vi "Autonomous_Load.vi"(0 "Number of Commands":i32, 5 "Subsystems":string[](array[string]), 7 "Commands":string[](array[string]), 9 "Inputs":string[][](array[string]), 11 "error in":errorcluster) -> (4 "Queue_Key":refnum<queue>, 10 "Autonomous_Queue":refnum<queue>, 15 "errror out":errorcluster)   [LabVIEW 2018]
uses:
  Autonomous Utilities/Queue_Key_Data.ctl
  Autonomous Utilities/Robot_Subsystems.ctl
  Subsytems/Drive/Drive_Notifier.ctl
  Subsytems/Drive/Drive_Control_Type.ctl
  Subsytems/Elevator/Elevator_Notifier.ctl
  Subsytems/Elevator/Elevator_Control_Type.ctl
  Subsytems/Elevator/Elevator_Enum_States.ctl
  Subsytems/Climb/Climb_Notifier.ctl
  Subsytems/Climb/Climb_Control_Type.ctl
  Subsytems/Intake_Ball/Intake_Ball_Notifier.ctl
  Subsytems/Intake_Ball/Intake_Ball_Control_Type.ctl
  Subsytems/Intake_Disc/Intake_Disc_Notifier.ctl
  Subsytems/Intake_Disc/Intake_Disc_Control_Type.ctl
  <vilib>/Rock Robotics/WPI/Solenoid/WPI_SolenoidValue.ctl
  Subsytems/Intake_Joint/Intake_Joint_Notifier.ctl
  Subsytems/Intake_Joint/Intake_Joint_Control_Type.ctl
  Subsytems/Intake_Joint/Intake_Joint_Enum_States.ctl
panel:
  in  "Intake_Disc_Control_Type":T1
  in  "Intake_Ball_Control_Type":T2
  in  "Set Position":T3=enum."High_Rocket_Hatch_Panel_Floor"
  in  "Intake_Joint_Control_Type":T4
  in  "Set_Position":T5=enum."High_Rocket_Hatch_Panel_Floor"
  in  "Elevator_Control_Type":T6
  in  "Climb_Control_Type":T7
  in  "Drive_Control_List":T8=enum."Write_FL_Position"
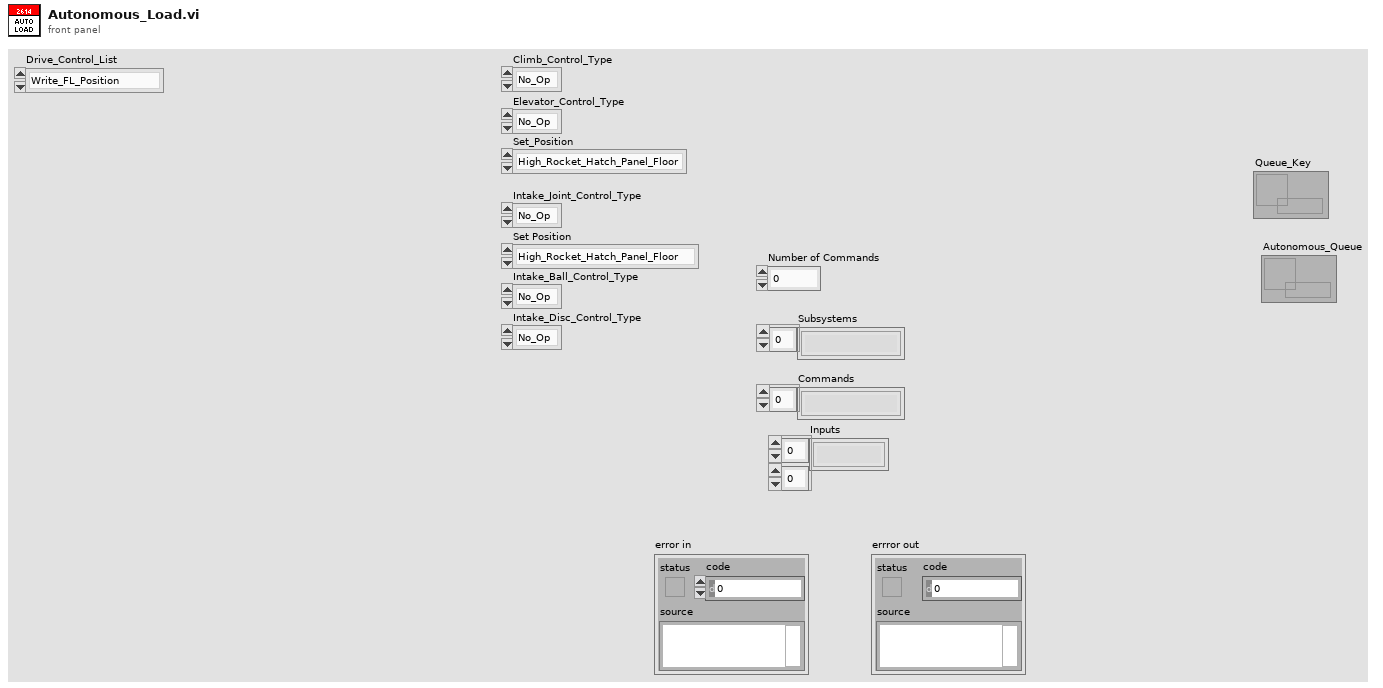
[diagram p1: front panel]
types:
  T1 = typedef "Intake_Disc_Control_Type.ctl" = enum16{"No_Op", "Manual_Disc_Toggle", "Disc_Toggle", "Manual_Press_Toggle", "Press_Toggle", "Acquire_Hatch", "Retract"}
  T2 = typedef "Intake_Ball_Control_Type.ctl" = enum16{"No_Op", "Manual_In", "Manual_Out", "In_Sensor_Stop", "Out_Teleop", "Out", "Stall"}
  T3 = typedef "Intake_Joint_Enum_States.ctl" = enum16{"Current_Position", "High_Rocket_Hatch_Panel_Floor", "High_Rocket_Hatch_Panel", "Mid_Rocket_Hatch_Panel_Floor", "Mid_Rocket_Hatch_Panel", "Low_Rocket_Hatch_Panel", "Cargo_Ship_Hatch_Panel", "Loading_Station_Hatch_Panel", "Ground_Pickup_Hatch_Panel", "High_Rocket_Cargo", "Mid_Rocket_Cargo", "Low_Rocket_Cargo", "Cargo_Ship_Cargo", "Loading_Station_Cargo", "Ground_Pickup_Cargo", "Depot_Pickup_Cargo", "Stow_Cargo", "Get_Hatch"}
  T4 = typedef "Intake_Joint_Control_Type.ctl" = enum16{"No_Op", "Manual_Joint_Up", "Manual_Joint_Down", "Manual_Position_Control", "Position_Control", "Position"}
  T5 = typedef "Elevator_Enum_States.ctl" = enum16{"Current_Position", "High_Rocket_Hatch_Panel_Floor", "High_Rocket_Hatch_Panel", "Mid_Rocket_Hatch_Panel_Floor", "Mid_Rocket_Hatch_Panel", "Low_Rocket_Hatch_Panel", "Cargo_Ship_Hatch_Panel", "Loading_Station_Hatch_Panel", "Ground_Pickup_Hatch_Panel", "High_Rocket_Cargo", "Mid_Rocket_Cargo", "Low_Rocket_Cargo", "Cargo_Ship_Cargo", "Loading_Station_Cargo", "Ground_Pickup_Cargo", "Depot_Pickup_Cargo", "Descend_Off_Platform", "Stow_Cargo"}
  T6 = typedef "Elevator_Control_Type.ctl" = enum16{"No_Op", "Shift", "Brake", "Manual_Elevator_Up", "Manual_Elevator_Down", "Manual_Climb_Up", "Manual_Climb_Down", "Manual_Position_Control", "Elevator_Retract", "Elevator_Extend", "Brake_In_Climb", "Position_Control", "Position", "Shift_Climb"}
  T7 = typedef "Climb_Control_Type.ctl" = enum16{"No_Op", "Brake", "Manual_Climb_Up", "Manual_Climb_Down", "Manual_Drive_Forward", "Manual_Drive_Backward", "Back_Wheels_Forward", "Lift_Retract", "Lift_Extend", "Extend_to_Second_Level", "Spin"}
  T8 = typedef "Drive_Control_Type.ctl" = enum16{"No_Op", "Write_FL_Position", "Write_FR_Position", "Write_BL_Position", "Write_BR_Position", "Set_Encoder_Positions", "Fieldcentric_PercentVBus", "Fieldcentric", "Robotcentric", "Reset_Gyro", "FR_Wheel", "FL_Wheel", "BR_Wheel", "BL_Wheel", "Drive_Onto_Platform", "Manual_Wheel_Control", "Distance", "Turn_To_Heading", "Turn_To_Target", "Drive_To_Target", "Zero", "Auto_Target", "Drive_Over_Platform", "Heading_Lock", "Time"}
  T9 = typedef "Queue_Key_Data.ctl" = cluster{"Operation Notifier":refnum<notifier>, "Subsystem":string, "Concurrent":bool}
  T10 = typedef "Robot_Subsystems.ctl" = cluster{"Drive Notifier":T11, "Elevator_Notifier":T12, "Climb_Notifier":T13, "Intake_Ball_Notifier":T14, "Intake_Disc_Notifier":T15, "Intake_Joint_Notifier":T17}
  T11 = typedef "Drive_Notifier.ctl" = cluster{"Drive Control List":T8, "Front/Back":dbl, "Left/Right":dbl, "Turn":dbl, "Test_Joy_Y":dbl, "Test_Joy_X":dbl, "Set Wheel Encoder Positions":bool, "Robotcentric":bool, "Reset Gyro":bool, "Rotate Front Right":bool, "Rotate Front Left":bool, "Rotate Back Right":bool, "Rotate Back Left":bool, "Write_Encoder_Positions":bool, "Climb_Advance":bool, "Parameter_One":dbl, "Parameter_Two":dbl, "Parameter_Three":dbl, "Parameter_Four":dbl, "Drive_Notifier":refnum<notifier>, "Step":i32, "Climb_Reverse":bool, "Auto_Target":bool}
  T12 = typedef "Elevator_Notifier.ctl" = cluster{"Elevator_Control_Type":T6, "Shift":bool, "Brake":bool, "Manual_Lift_Up":bool, "Manual_Lift_Down":bool, "Climb_Advance":bool, "Climb_Reverse":bool, "Low_Rocket":bool, "Mid_Rocket":bool, "High_Rocket":bool, "Cargo_Ship":bool, "Hatch_Floor":bool, "Cargo_Floor":bool, "HP_Hatch":bool, "HP_Cargo":bool, "Depot_Cargo":bool, "Stow":bool, "Set_Position":T5, "Intake_Mode":bool, "Climb_Distance":dbl, "Level_Two":bool, "Parameter_One":dbl, "Parameter_Two":dbl, "Parameter_Three":dbl, "Step":i32, "Elevator_Notifier":refnum<notifier>, "Brake_State":bool, "Shift_State":bool}
  T13 = typedef "Climb_Notifier.ctl" = cluster{"Climb_Control_Type":T7, "Brake":bool, "Manual_Climb_Up":bool, "Manual_Drive_Forward":bool, "Manual_Drive_Backward":bool, "Manual_Climb_Down":bool, "Climb_Advance":bool, "Climb_Reverse":bool, "Parameter_One":dbl, "Parameter_Two":dbl, "Parameter_Three":dbl, "Step":i32, "Climb_Notifier":refnum<notifier>, "Climb_Distance":dbl, "Level_Two":bool, "Brake_State":bool, "Toggle_Servo":bool}
  T14 = typedef "Intake_Ball_Notifier.ctl" = cluster{"Intake_Ball_Control_Type":T2, "Manual_In":bool, "Manual_Out":bool, "Ball_In":bool, "Ball_Out":bool, "Parameter_One":dbl, "Parameter_Two":dbl, "Parameter_Three":dbl, "Step":i32, "Ball_Notifier":refnum<notifier>}
  T15 = typedef "Intake_Disc_Notifier.ctl" = cluster{"Intake_Disc_Control_Type":T1, "Manual_Disc_Toggle":bool, "Disc_Toggle":bool, "Disc_Toggle_State":bool, "Manual_Press_Toggle":bool, "Disc_Press_State":bool, "Press_Toggle":bool, "Press_Pnuematic":T16, "Disc_Pnuematic":T16, "Disc_Notifier":refnum<notifier>, "Step":i32}
  T16 = typedef "WPI_SolenoidValue.ctl" = enum16{"Off", "On", "Forward", "Reverse"}
  T17 = typedef "Intake_Joint_Notifier.ctl" = cluster{"Intake_Joint_Control_Type":T4, "Manual_Joint_Up":bool, "Manual_Joint_Down":bool, "Low_Rocket":bool, "Mid_Rocket":bool, "High_Rocket":bool, "Cargo_Ship":bool, "Hatch_Floor":bool, "Cargo_Floor":bool, "HP_Hatch":bool, "HP_Cargo":bool, "Depot_Cargo":bool, "Stow":bool, "Intake_Mode":bool, "Set Position":T3, "Parameter_One":dbl, "Parameter_Two":dbl, "Parameter_Three":dbl, "Step":i32, "Joint_Notifier":refnum<notifier>}
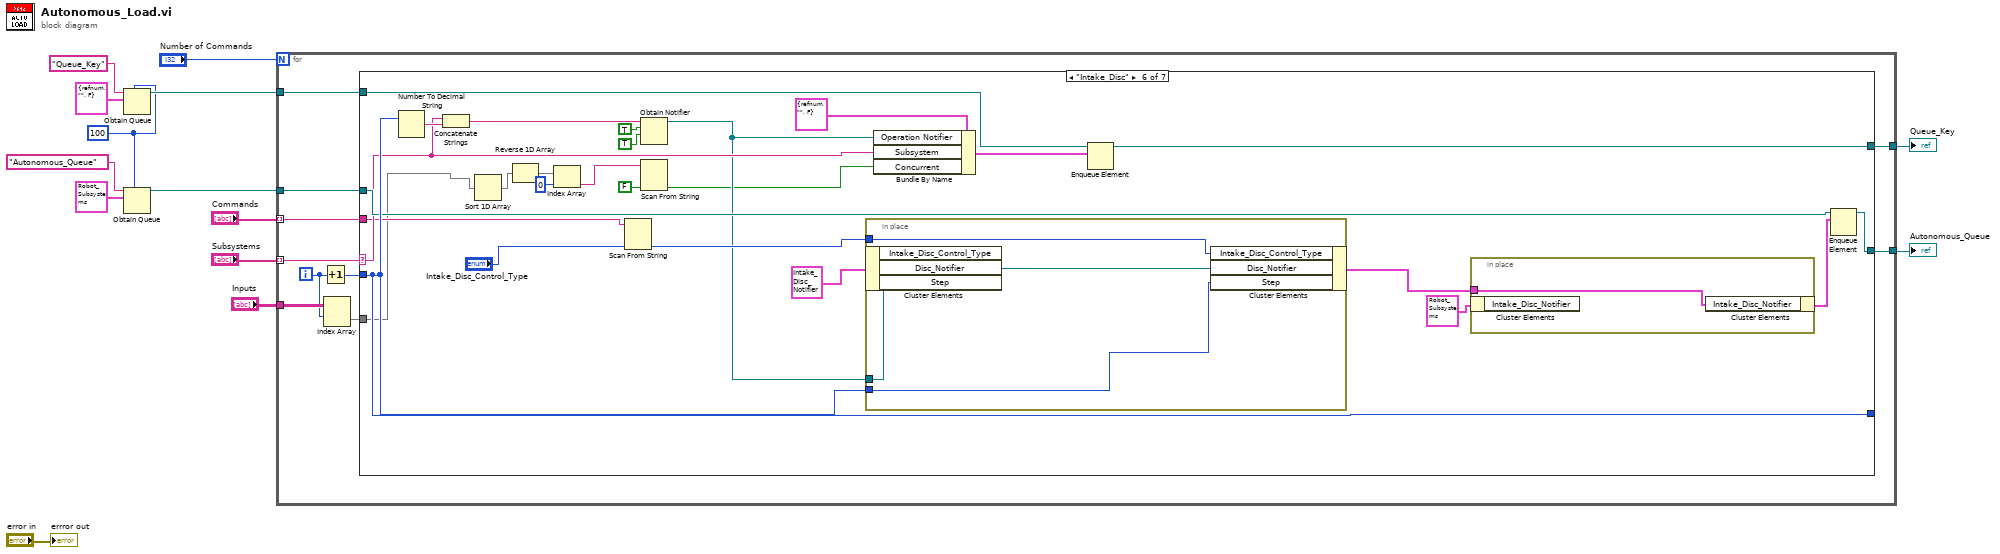
[diagram p0: block diagram]
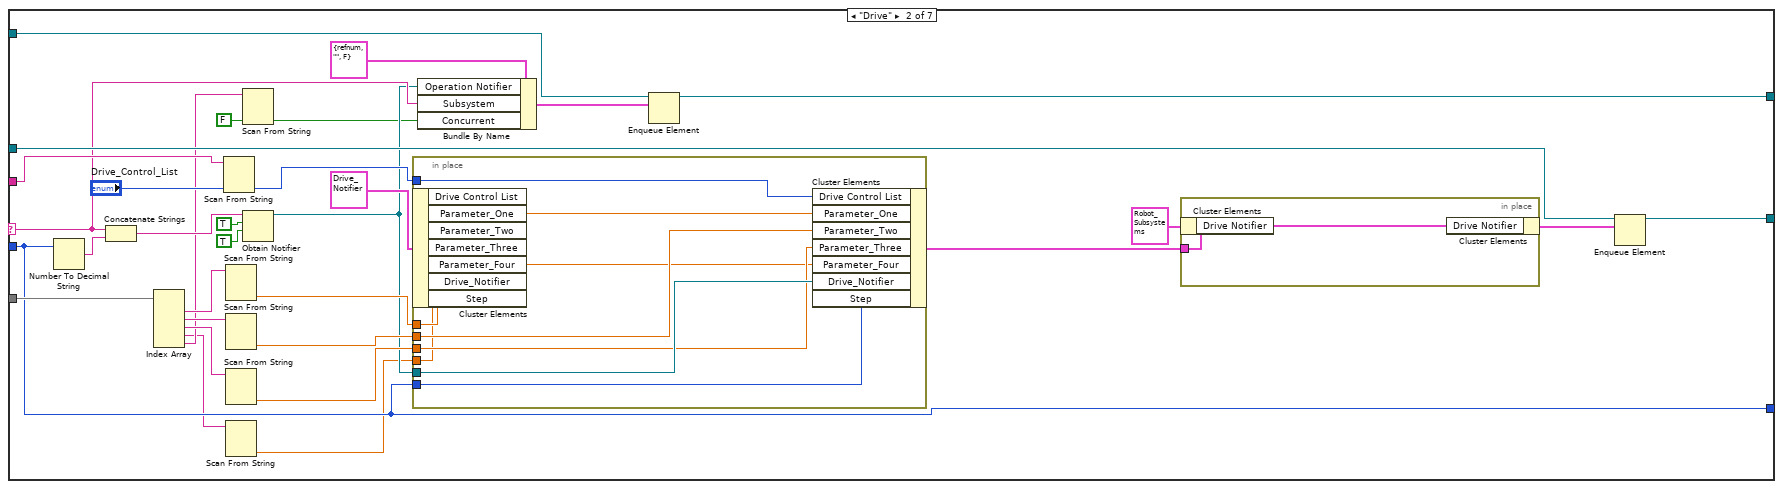
[diagram p3: hidden frame]
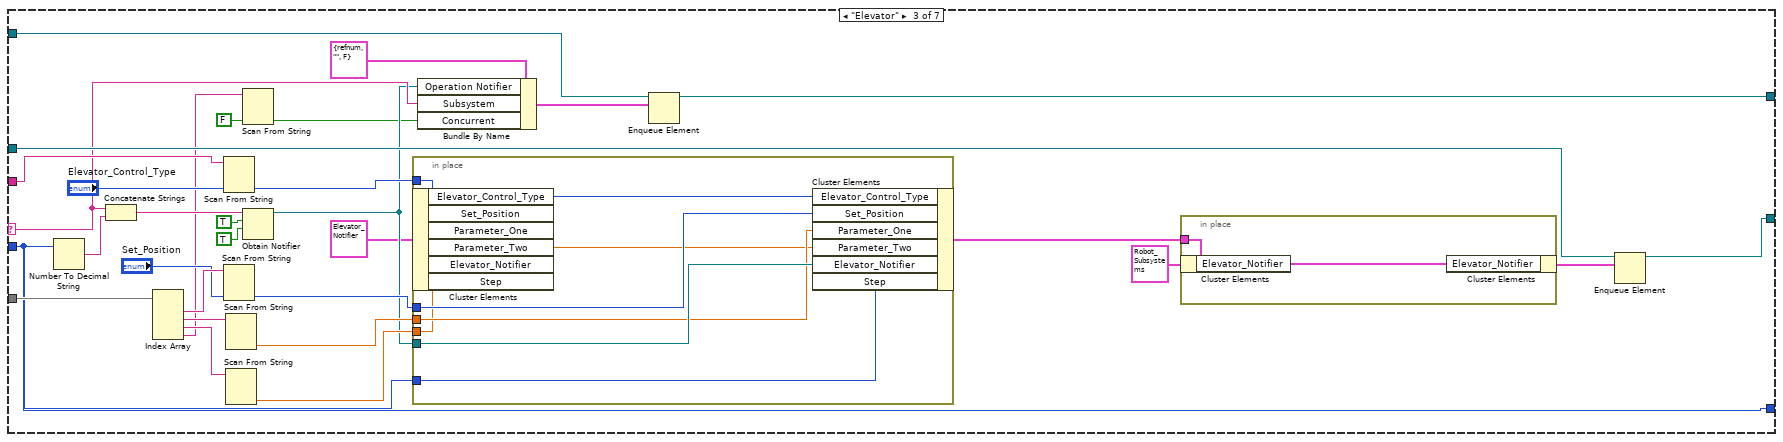
[diagram p4: hidden frame]
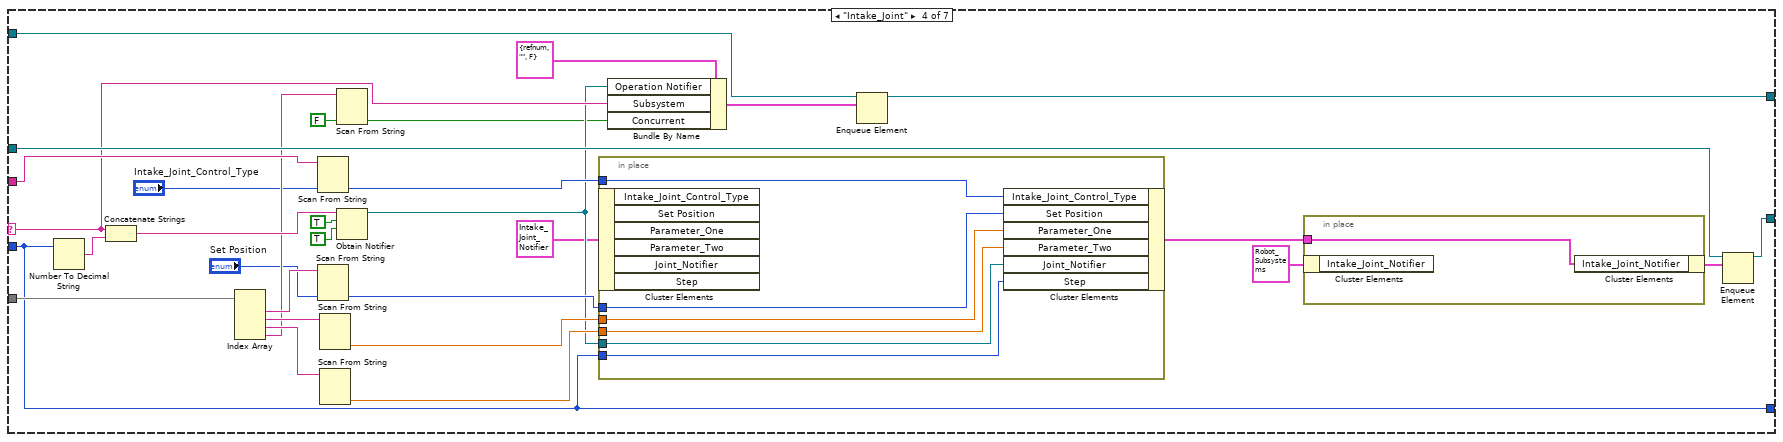
[diagram p5: hidden frame]
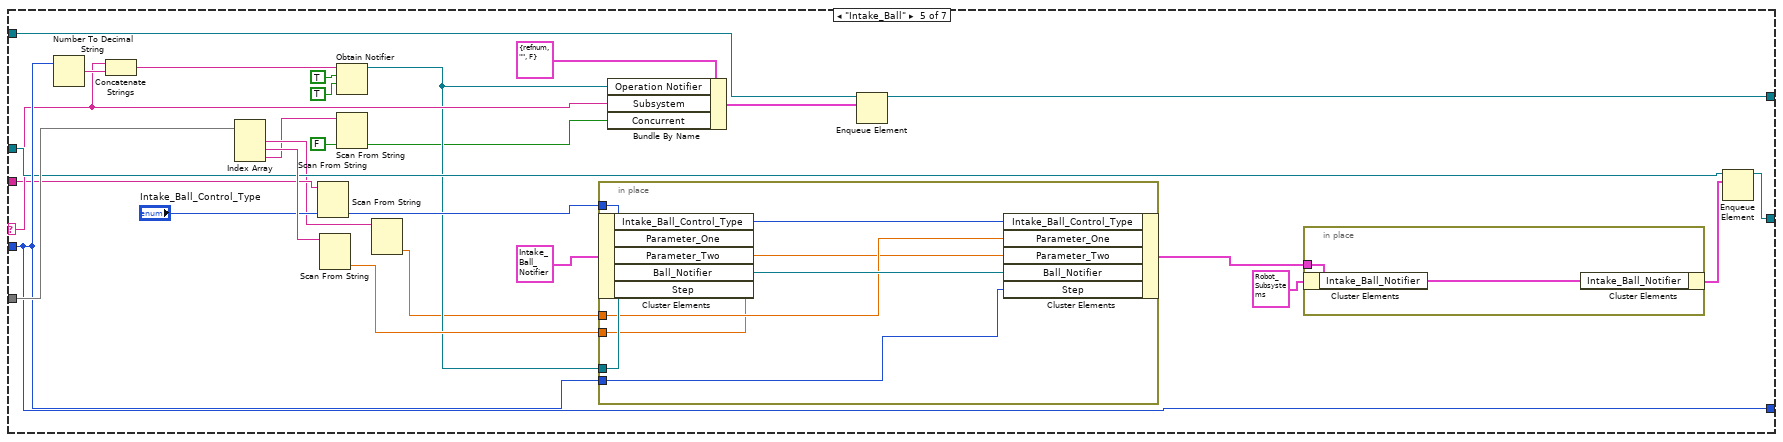
[diagram p6: hidden frame]
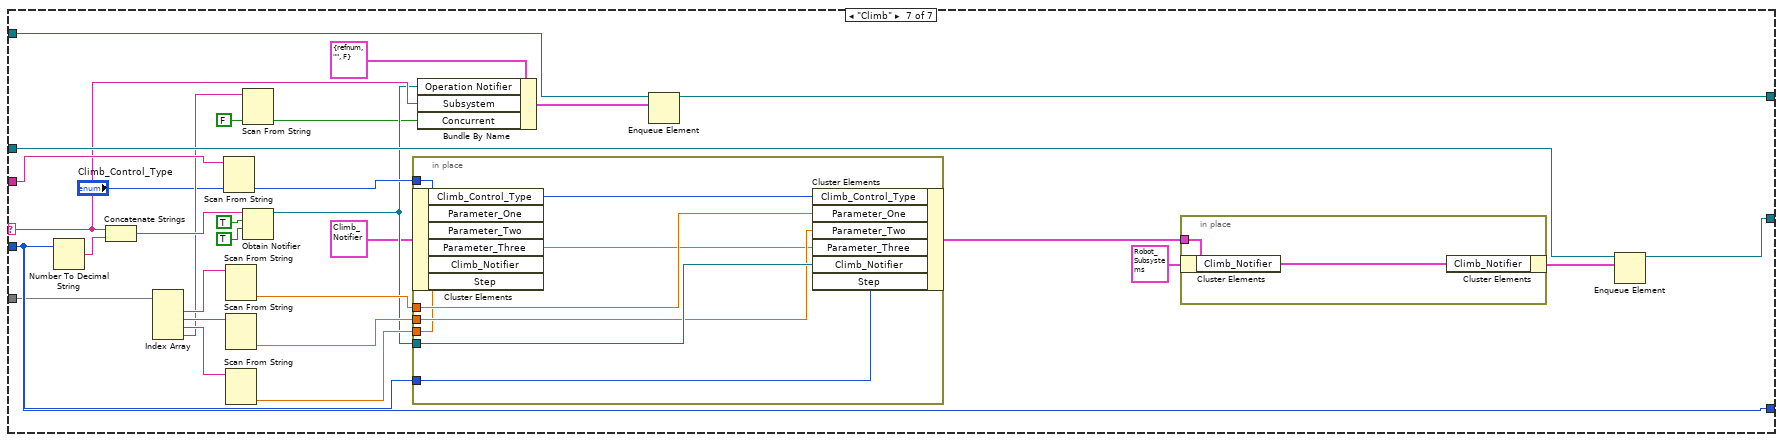
[diagram p7: hidden frame]
diagram:
  w6 = 100 ("max queue size (-1, unlimited)")
  n1 = Obtain Queue(max queue size (-1, unlimited)=w6, name (unnamed)="Queue_Key", element data type=T9 {"Operation Notifier"=refnum, "Subsystem"="", "Concurrent"=FALSE} ("Queue Key Data")) -> (queue out=w12:refnum<queue>)  [unwired: 2 in, 2 out]
  n2 = Obtain Queue(max queue size (-1, unlimited)=w6, name (unnamed)="Autonomous_Queue", element data type=T10 {"Drive Notifier"={"Drive Control List"=enum."No_Op", "Front/Back"=0.0, "Left/Right"=0.0, "Turn"=0.0, "Test_Joy_Y"=0.0, "Test_Joy_X"=0.0, "Set Wheel Encoder Positions"=FALSE, "Robotcentric"=FALSE, "Reset Gyro"=FALSE, "Rotate Front Right"=FALSE, "Rotate Front Left"=FALSE, "Rotate Back Right"=FALSE, "Rotate Back Left"=FALSE, "Write_Encoder_Positions"=FALSE, "Climb_Advance"=FALSE, "Parameter_One"=0.0, "Parameter_Two"=0.0, "Parameter_Three"=0.0, "Parameter_Four"=0.0, "Drive_Notifier"=refnum, "Step"=0, "Climb_Reverse"=FALSE, "Auto_Target"=FALSE}, "Elevator_Notifier"={"Elevator_Control_Type"=enum."No_Op", "Shift"=FALSE, "Brake"=FALSE, "Manual_Lift_Up"=FALSE, "Manual_Lift_Down"=FALSE, "Climb_Advance"=FALSE, "Climb_Reverse"=FALSE, "Low_Rocket"=FALSE, "Mid_Rocket"=FALSE, "High_Rocket"=FALSE, "Cargo_Ship"=FALSE, "Hatch_Floor"=FALSE, "Cargo_Floor"=FALSE, "HP_Hatch"=FALSE, "HP_Cargo"=FALSE, "Depot_Cargo"=FALSE, "Stow"=FALSE, "Set_Position"=enum."High_Rocket_Hatch_Panel", "Intake_Mode"=FALSE, "Climb_Distance"=0.0, "Level_Two"=FALSE, "Parameter_One"=0.0, "Parameter_Two"=0.0, "Parameter_Three"=0.0, "Step"=0, "Elevator_Notifier"=refnum, "Brake_State"=FALSE, "Shift_State"=FALSE}, "Climb_Notifier"={"Climb_Control_Type"=enum."No_Op", "Brake"=FALSE, "Manual_Climb_Up"=FALSE, "Manual_Drive_Forward"=FALSE, "Manual_Drive_Backward"=FALSE, "Manual_Climb_Down"=FALSE, "Climb_Advance"=FALSE, "Climb_Reverse"=FALSE, "Parameter_One"=0.0, "Parameter_Two"=0.0, "Parameter_Three"=0.0, "Step"=0, "Climb_Notifier"=refnum, "Climb_Distance"=0.0, "Level_Two"=FALSE, "Brake_State"=FALSE, "Toggle_Servo"=FALSE}, "Intake_Ball_Notifier"={"Intake_Ball_Control_Type"=enum."No_Op", "Manual_In"=FALSE, "Manual_Out"=FALSE, "Ball_In"=FALSE, "Ball_Out"=FALSE, "Parameter_One"=0.0, "Parameter_Two"=0.0, "Parameter_Three"=0.0, "Step"=0, "Ball_Notifier"=refnum}, "Intake_Disc_Notifier"={"Intake_Disc_Control_Type"=enum."No_Op", "Manual_Disc_Toggle"=FALSE, "Disc_Toggle"=FALSE, "Disc_Toggle_State"=FALSE, "Manual_Press_Toggle"=FALSE, "Disc_Press_State"=FALSE, "Press_Toggle"=FALSE, "Press_Pnuematic"=enum."Forward", "Disc_Pnuematic"=enum."Forward", "Disc_Notifier"=refnum, "Step"=0}, "Intake_Joint_Notifier"={"Intake_Joint_Control_Type"=enum."No_Op", "Manual_Joint_Up"=FALSE, "Manual_Joint_Down"=FALSE, "Low_Rocket"=FALSE, "Mid_Rocket"=FALSE, "High_Rocket"=FALSE, "Cargo_Ship"=FALSE, "Hatch_Floor"=FALSE, "Cargo_Floor"=FALSE, "HP_Hatch"=FALSE, "HP_Cargo"=FALSE, "Depot_Cargo"=FALSE, "Stow"=FALSE, "Intake_Mode"=FALSE, "Set Position"=enum."High_Rocket_Hatch_Panel", "Parameter_One"=0.0, "Parameter_Two"=0.0, "Parameter_Three"=0.0, "Step"=0, "Joint_Notifier"=refnum}} ("Robot Subsytems")) -> (queue out=w7:refnum<queue>)  [unwired: 2 in, 2 out]
  n3 = for {
    N: "Number of Commands" -> [_]
    tunnel: w12 -> [w24]
    tunnel: "Subsystems" -> [w23] mode=indexing
    tunnel: "Commands" -> [w22] mode=indexing
    tunnel: "Inputs" -> [w18]
    tunnel: [w21] -> w3
    tunnel: w7 -> [w20]
    tunnel: [w15] -> w2
    i -> [w16]
    n4 = Increment(x=w16) -> (x+1=w19:i32)
    n5 = Index Array(array=w18, index (row)=w16) -> (element=w17:string[])  [unwired: 1 in]
    n6 = case shown="\"Intake_Disc\"" w23 {
      selector: w23 -> [_ w35 w76 w114 w154 w190 w217]
      tunnel: w24 -> [w26 w38 w79 w117 w157 w193 w220]
      tunnel: w22 -> [_ w54 w94 w132 w147 w185 w234]
      tunnel: [w27 w39 w80 w118 w158 w194 w221] -> w15
      tunnel: [w26 w31 w72 w110 w150 w186 w212] -> w21
      tunnel: w20 -> [w27 w43 w84 w122 w162 w198 w225]
      tunnel: w19 -> [w25 w50 w91 w129 w166 w200 w232]
      tunnel: [w25 w50 w91 w129 w166 w200 w232] -> _
      tunnel: w17 -> [_ w51 w92 w130 w167 w180 w209]
      frame "No Op", Default {
      }
      frame "Drive" {
        n7 = Number To Decimal String(number=w50) -> (decimal integer string=w57:string)  [unwired: 1 in]
        n8 = Concatenate Strings(w35, w57) -> (w56:string)
        n9 = Index Array(array=w51) -> (element #1=w49:string, element #2=w47:string, element #3=w44:string, element #4=w29:string, element #5=w30:string)  [unwired: 5 in]
        n10 = Scan From String(input string=w54, default 1="Drive_Control_List") -> (output 1=w52:T8)  [unwired: 3 in, 3 out]
        n11 = Scan From String(input string=w49) -> (output 1=w48:dbl)  [unwired: 4 in, 3 out]
        n12 = Scan From String(input string=w47) -> (output 1=w46:dbl)  [unwired: 4 in, 3 out]
        n13 = Scan From String(input string=w44) -> (output 1=w45:dbl)  [unwired: 4 in, 3 out]
        n14 = Scan From String(input string=w29) -> (output 1=w28:dbl)  [unwired: 4 in, 3 out]
        n15 = Scan From String(input string=w30, default 1=FALSE) -> (output 1=w32:bool)  [unwired: 3 in, 3 out]
        n16 = Obtain Notifier(name (unnamed)=w56, notification data type=TRUE ("create if not found? (T)"), create if not found? (T)=TRUE) -> (notifier out=w34:refnum<notifier>)  [unwired: 1 in, 2 out]
        n17 = in-place {
          in-place-border: w52 -> [w67]
          in-place-border: w34 -> [w66]
          in-place-border: w50 -> [w65]
          in-place-border: w48 -> [w64]
          in-place-border: w46 -> [w63]
          in-place-border: w45 -> [w62]
          in-place-border: w28 -> [w61]
          n18 = in-place-cluster #1(T11 {"Drive Control List"=enum."No_Op", "Front/Back"=0.0, "Left/Right"=0.0, "Turn"=0.0, "Test_Joy_Y"=0.0, "Test_Joy_X"=0.0, "Set Wheel Encoder Positions"=FALSE, "Robotcentric"=FALSE, "Reset Gyro"=FALSE, "Rotate Front Right"=FALSE, "Rotate Front Left"=FALSE, "Rotate Back Right"=FALSE, "Rotate Back Left"=FALSE, "Write_Encoder_Positions"=FALSE, "Climb_Advance"=FALSE, "Parameter_One"=0.0, "Parameter_Two"=0.0, "Parameter_Three"=0.0, "Parameter_Four"=0.0, "Drive_Notifier"=refnum, "Step"=0, "Climb_Reverse"=FALSE, "Auto_Target"=FALSE} ("Drive Notifier")) -> ()  [unwired: 7 out]
          n19 = in-place-cluster #1("Drive Control List"=w67, "Parameter_One"=w64, "Parameter_Two"=w63, "Parameter_Three"=w62, "Parameter_Four"=w61, "Drive_Notifier"=w66, "Step"=w65) -> (w41:T11)
        }
        n20 = Bundle By Name(cluster=T9 {"Operation Notifier"=refnum, "Subsystem"="", "Concurrent"=FALSE} ("Queue Key Data"), "Operation Notifier"=w34, "Subsystem"=w35, "Concurrent"=w32) -> (w37:T9)
        n21 = Enqueue Element(queue=w38, element=w37) -> (queue out=w31:refnum<queue>)  [unwired: 2 in, 2 out]
        n22 = in-place {
          in-place-border: w41 -> [w60]
          n23 = in-place-cluster #2(T10 {"Drive Notifier"={"Drive Control List"=enum."No_Op", "Front/Back"=0.0, "Left/Right"=0.0, "Turn"=0.0, "Test_Joy_Y"=0.0, "Test_Joy_X"=0.0, "Set Wheel Encoder Positions"=FALSE, "Robotcentric"=FALSE, "Reset Gyro"=FALSE, "Rotate Front Right"=FALSE, "Rotate Front Left"=FALSE, "Rotate Back Right"=FALSE, "Rotate Back Left"=FALSE, "Write_Encoder_Positions"=FALSE, "Climb_Advance"=FALSE, "Parameter_One"=0.0, "Parameter_Two"=0.0, "Parameter_Three"=0.0, "Parameter_Four"=0.0, "Drive_Notifier"=refnum, "Step"=0, "Climb_Reverse"=FALSE, "Auto_Target"=FALSE}, "Elevator_Notifier"={"Elevator_Control_Type"=enum."No_Op", "Shift"=FALSE, "Brake"=FALSE, "Manual_Lift_Up"=FALSE, "Manual_Lift_Down"=FALSE, "Climb_Advance"=FALSE, "Climb_Reverse"=FALSE, "Low_Rocket"=FALSE, "Mid_Rocket"=FALSE, "High_Rocket"=FALSE, "Cargo_Ship"=FALSE, "Hatch_Floor"=FALSE, "Cargo_Floor"=FALSE, "HP_Hatch"=FALSE, "HP_Cargo"=FALSE, "Depot_Cargo"=FALSE, "Stow"=FALSE, "Set_Position"=enum."High_Rocket_Hatch_Panel", "Intake_Mode"=FALSE, "Climb_Distance"=0.0, "Level_Two"=FALSE, "Parameter_One"=0.0, "Parameter_Two"=0.0, "Parameter_Three"=0.0, "Step"=0, "Elevator_Notifier"=refnum, "Brake_State"=FALSE, "Shift_State"=FALSE}, "Climb_Notifier"={"Climb_Control_Type"=enum."No_Op", "Brake"=FALSE, "Manual_Climb_Up"=FALSE, "Manual_Drive_Forward"=FALSE, "Manual_Drive_Backward"=FALSE, "Manual_Climb_Down"=FALSE, "Climb_Advance"=FALSE, "Climb_Reverse"=FALSE, "Parameter_One"=0.0, "Parameter_Two"=0.0, "Parameter_Three"=0.0, "Step"=0, "Climb_Notifier"=refnum, "Climb_Distance"=0.0, "Level_Two"=FALSE, "Brake_State"=FALSE, "Toggle_Servo"=FALSE}, "Intake_Ball_Notifier"={"Intake_Ball_Control_Type"=enum."No_Op", "Manual_In"=FALSE, "Manual_Out"=FALSE, "Ball_In"=FALSE, "Ball_Out"=FALSE, "Parameter_One"=0.0, "Parameter_Two"=0.0, "Parameter_Three"=0.0, "Step"=0, "Ball_Notifier"=refnum}, "Intake_Disc_Notifier"={"Intake_Disc_Control_Type"=enum."No_Op", "Manual_Disc_Toggle"=FALSE, "Disc_Toggle"=FALSE, "Disc_Toggle_State"=FALSE, "Manual_Press_Toggle"=FALSE, "Disc_Press_State"=FALSE, "Press_Toggle"=FALSE, "Press_Pnuematic"=enum."Forward", "Disc_Pnuematic"=enum."Forward", "Disc_Notifier"=refnum, "Step"=0}, "Intake_Joint_Notifier"={"Intake_Joint_Control_Type"=enum."No_Op", "Manual_Joint_Up"=FALSE, "Manual_Joint_Down"=FALSE, "Low_Rocket"=FALSE, "Mid_Rocket"=FALSE, "High_Rocket"=FALSE, "Cargo_Ship"=FALSE, "Hatch_Floor"=FALSE, "Cargo_Floor"=FALSE, "HP_Hatch"=FALSE, "HP_Cargo"=FALSE, "Depot_Cargo"=FALSE, "Stow"=FALSE, "Intake_Mode"=FALSE, "Set Position"=enum."High_Rocket_Hatch_Panel", "Parameter_One"=0.0, "Parameter_Two"=0.0, "Parameter_Three"=0.0, "Step"=0, "Joint_Notifier"=refnum}} ("Robot Subsytems")) -> ()  [unwired: 1 out]
          n24 = in-place-cluster #2("Drive Notifier"=w60) -> (w40:T10)
        }
        n25 = Enqueue Element(queue=w43, element=w40) -> (queue out=w39:refnum<queue>)  [unwired: 2 in, 2 out]
      }
      frame "Elevator" {
        n26 = Number To Decimal String(number=w91) -> (decimal integer string=w96:string)  [unwired: 1 in]
        n27 = Concatenate Strings(w76, w96) -> (w95:string)
        n28 = Index Array(array=w92) -> (element #1=w90:string, element #2=w88:string, element #3=w85:string, element #4=w68:string)  [unwired: 4 in]
        n29 = Scan From String(input string=w94, default 1="Elevator_Control_Type") -> (output 1=w93:T6)  [unwired: 3 in, 3 out]
        n30 = Scan From String(input string=w90, default 1="Set_Position") -> (output 1=w89:T5)  [unwired: 3 in, 3 out]
        n31 = Scan From String(input string=w88) -> (output 1=w87:dbl)  [unwired: 4 in, 3 out]
        n32 = Scan From String(input string=w85) -> (output 1=w86:dbl)  [unwired: 4 in, 3 out]
        n33 = Scan From String(input string=w68, default 1=FALSE) -> (output 1=w73:bool)  [unwired: 3 in, 3 out]
        n34 = Obtain Notifier(name (unnamed)=w95, notification data type=TRUE ("create if not found? (T)"), create if not found? (T)=TRUE) -> (notifier out=w75:refnum<notifier>)  [unwired: 1 in, 2 out]
        n35 = in-place {
          in-place-border: w93 -> [w105]
          in-place-border: w75 -> [w103]
          in-place-border: w91 -> [w104]
          in-place-border: w89 -> [w102]
          in-place-border: w87 -> [w101]
          in-place-border: w86 -> [w100]
          n36 = in-place-cluster #3(T12 {"Elevator_Control_Type"=enum."No_Op", "Shift"=FALSE, "Brake"=FALSE, "Manual_Lift_Up"=FALSE, "Manual_Lift_Down"=FALSE, "Climb_Advance"=FALSE, "Climb_Reverse"=FALSE, "Low_Rocket"=FALSE, "Mid_Rocket"=FALSE, "High_Rocket"=FALSE, "Cargo_Ship"=FALSE, "Hatch_Floor"=FALSE, "Cargo_Floor"=FALSE, "HP_Hatch"=FALSE, "HP_Cargo"=FALSE, "Depot_Cargo"=FALSE, "Stow"=FALSE, "Set_Position"=enum."High_Rocket_Hatch_Panel", "Intake_Mode"=FALSE, "Climb_Distance"=0.0, "Level_Two"=FALSE, "Parameter_One"=0.0, "Parameter_Two"=0.0, "Parameter_Three"=0.0, "Step"=0, "Elevator_Notifier"=refnum, "Brake_State"=FALSE, "Shift_State"=FALSE} ("Elevator_Notifier")) -> ()  [unwired: 6 out]
          n37 = in-place-cluster #3("Elevator_Control_Type"=w105, "Set_Position"=w102, "Parameter_One"=w101, "Parameter_Two"=w100, "Elevator_Notifier"=w103, "Step"=w104) -> (w82:T12)
        }
        n38 = Bundle By Name(cluster=T9 {"Operation Notifier"=refnum, "Subsystem"="", "Concurrent"=FALSE} ("Queue Key Data"), "Operation Notifier"=w75, "Subsystem"=w76, "Concurrent"=w73) -> (w78:T9)
        n39 = Enqueue Element(queue=w79, element=w78) -> (queue out=w72:refnum<queue>)  [unwired: 2 in, 2 out]
        n40 = in-place {
          in-place-border: w82 -> [w99]
          n41 = in-place-cluster #4(T10 {"Drive Notifier"={"Drive Control List"=enum."No_Op", "Front/Back"=0.0, "Left/Right"=0.0, "Turn"=0.0, "Test_Joy_Y"=0.0, "Test_Joy_X"=0.0, "Set Wheel Encoder Positions"=FALSE, "Robotcentric"=FALSE, "Reset Gyro"=FALSE, "Rotate Front Right"=FALSE, "Rotate Front Left"=FALSE, "Rotate Back Right"=FALSE, "Rotate Back Left"=FALSE, "Write_Encoder_Positions"=FALSE, "Climb_Advance"=FALSE, "Parameter_One"=0.0, "Parameter_Two"=0.0, "Parameter_Three"=0.0, "Parameter_Four"=0.0, "Drive_Notifier"=refnum, "Step"=0, "Climb_Reverse"=FALSE, "Auto_Target"=FALSE}, "Elevator_Notifier"={"Elevator_Control_Type"=enum."No_Op", "Shift"=FALSE, "Brake"=FALSE, "Manual_Lift_Up"=FALSE, "Manual_Lift_Down"=FALSE, "Climb_Advance"=FALSE, "Climb_Reverse"=FALSE, "Low_Rocket"=FALSE, "Mid_Rocket"=FALSE, "High_Rocket"=FALSE, "Cargo_Ship"=FALSE, "Hatch_Floor"=FALSE, "Cargo_Floor"=FALSE, "HP_Hatch"=FALSE, "HP_Cargo"=FALSE, "Depot_Cargo"=FALSE, "Stow"=FALSE, "Set_Position"=enum."High_Rocket_Hatch_Panel", "Intake_Mode"=FALSE, "Climb_Distance"=0.0, "Level_Two"=FALSE, "Parameter_One"=0.0, "Parameter_Two"=0.0, "Parameter_Three"=0.0, "Step"=0, "Elevator_Notifier"=refnum, "Brake_State"=FALSE, "Shift_State"=FALSE}, "Climb_Notifier"={"Climb_Control_Type"=enum."No_Op", "Brake"=FALSE, "Manual_Climb_Up"=FALSE, "Manual_Drive_Forward"=FALSE, "Manual_Drive_Backward"=FALSE, "Manual_Climb_Down"=FALSE, "Climb_Advance"=FALSE, "Climb_Reverse"=FALSE, "Parameter_One"=0.0, "Parameter_Two"=0.0, "Parameter_Three"=0.0, "Step"=0, "Climb_Notifier"=refnum, "Climb_Distance"=0.0, "Level_Two"=FALSE, "Brake_State"=FALSE, "Toggle_Servo"=FALSE}, "Intake_Ball_Notifier"={"Intake_Ball_Control_Type"=enum."No_Op", "Manual_In"=FALSE, "Manual_Out"=FALSE, "Ball_In"=FALSE, "Ball_Out"=FALSE, "Parameter_One"=0.0, "Parameter_Two"=0.0, "Parameter_Three"=0.0, "Step"=0, "Ball_Notifier"=refnum}, "Intake_Disc_Notifier"={"Intake_Disc_Control_Type"=enum."No_Op", "Manual_Disc_Toggle"=FALSE, "Disc_Toggle"=FALSE, "Disc_Toggle_State"=FALSE, "Manual_Press_Toggle"=FALSE, "Disc_Press_State"=FALSE, "Press_Toggle"=FALSE, "Press_Pnuematic"=enum."Forward", "Disc_Pnuematic"=enum."Forward", "Disc_Notifier"=refnum, "Step"=0}, "Intake_Joint_Notifier"={"Intake_Joint_Control_Type"=enum."No_Op", "Manual_Joint_Up"=FALSE, "Manual_Joint_Down"=FALSE, "Low_Rocket"=FALSE, "Mid_Rocket"=FALSE, "High_Rocket"=FALSE, "Cargo_Ship"=FALSE, "Hatch_Floor"=FALSE, "Cargo_Floor"=FALSE, "HP_Hatch"=FALSE, "HP_Cargo"=FALSE, "Depot_Cargo"=FALSE, "Stow"=FALSE, "Intake_Mode"=FALSE, "Set Position"=enum."High_Rocket_Hatch_Panel", "Parameter_One"=0.0, "Parameter_Two"=0.0, "Parameter_Three"=0.0, "Step"=0, "Joint_Notifier"=refnum}} ("Robot Subsytems")) -> ()  [unwired: 1 out]
          n42 = in-place-cluster #4("Elevator_Notifier"=w99) -> (w81:T10)
        }
        n43 = Enqueue Element(queue=w84, element=w81) -> (queue out=w80:refnum<queue>)  [unwired: 2 in, 2 out]
      }
      frame "Intake_Joint" {
        n44 = Number To Decimal String(number=w129) -> (decimal integer string=w134:string)  [unwired: 1 in]
        n45 = Concatenate Strings(w114, w134) -> (w133:string)
        n46 = Index Array(array=w130) -> (element #1=w128:string, element #2=w126:string, element #3=w123:string, element #4=w109:string)  [unwired: 4 in]
        n47 = Scan From String(input string=w132, default 1="Intake_Joint_Control_Type") -> (output 1=w131:T4)  [unwired: 3 in, 3 out]
        n48 = Scan From String(input string=w128, default 1="Set Position") -> (output 1=w127:T3)  [unwired: 3 in, 3 out]
        n49 = Scan From String(input string=w126) -> (output 1=w125:dbl)  [unwired: 4 in, 3 out]
        n50 = Scan From String(input string=w123) -> (output 1=w124:dbl)  [unwired: 4 in, 3 out]
        n51 = Scan From String(input string=w109, default 1=FALSE) -> (output 1=w111:bool)  [unwired: 3 in, 3 out]
        n52 = Obtain Notifier(name (unnamed)=w133, notification data type=TRUE ("create if not found? (T)"), create if not found? (T)=TRUE) -> (notifier out=w113:refnum<notifier>)  [unwired: 1 in, 2 out]
        n53 = in-place {
          in-place-border: w131 -> [w143]
          in-place-border: w113 -> [w141]
          in-place-border: w129 -> [w142]
          in-place-border: w127 -> [w140]
          in-place-border: w125 -> [w139]
          in-place-border: w124 -> [w138]
          n54 = in-place-cluster #5(T17 {"Intake_Joint_Control_Type"=enum."No_Op", "Manual_Joint_Up"=FALSE, "Manual_Joint_Down"=FALSE, "Low_Rocket"=FALSE, "Mid_Rocket"=FALSE, "High_Rocket"=FALSE, "Cargo_Ship"=FALSE, "Hatch_Floor"=FALSE, "Cargo_Floor"=FALSE, "HP_Hatch"=FALSE, "HP_Cargo"=FALSE, "Depot_Cargo"=FALSE, "Stow"=FALSE, "Intake_Mode"=FALSE, "Set Position"=enum."High_Rocket_Hatch_Panel", "Parameter_One"=0.0, "Parameter_Two"=0.0, "Parameter_Three"=0.0, "Step"=0, "Joint_Notifier"=refnum} ("Intake_Joint_Notifier")) -> ()  [unwired: 6 out]
          n55 = in-place-cluster #5("Intake_Joint_Control_Type"=w143, "Set Position"=w140, "Parameter_One"=w139, "Parameter_Two"=w138, "Joint_Notifier"=w141, "Step"=w142) -> (w120:T17)
        }
        n56 = Bundle By Name(cluster=T9 {"Operation Notifier"=refnum, "Subsystem"="", "Concurrent"=FALSE} ("Queue Key Data"), "Operation Notifier"=w113, "Subsystem"=w114, "Concurrent"=w111) -> (w116:T9)
        n57 = Enqueue Element(queue=w117, element=w116) -> (queue out=w110:refnum<queue>)  [unwired: 2 in, 2 out]
        n58 = in-place {
          in-place-border: w120 -> [w137]
          n59 = in-place-cluster #6(T10 {"Drive Notifier"={"Drive Control List"=enum."No_Op", "Front/Back"=0.0, "Left/Right"=0.0, "Turn"=0.0, "Test_Joy_Y"=0.0, "Test_Joy_X"=0.0, "Set Wheel Encoder Positions"=FALSE, "Robotcentric"=FALSE, "Reset Gyro"=FALSE, "Rotate Front Right"=FALSE, "Rotate Front Left"=FALSE, "Rotate Back Right"=FALSE, "Rotate Back Left"=FALSE, "Write_Encoder_Positions"=FALSE, "Climb_Advance"=FALSE, "Parameter_One"=0.0, "Parameter_Two"=0.0, "Parameter_Three"=0.0, "Parameter_Four"=0.0, "Drive_Notifier"=refnum, "Step"=0, "Climb_Reverse"=FALSE, "Auto_Target"=FALSE}, "Elevator_Notifier"={"Elevator_Control_Type"=enum."No_Op", "Shift"=FALSE, "Brake"=FALSE, "Manual_Lift_Up"=FALSE, "Manual_Lift_Down"=FALSE, "Climb_Advance"=FALSE, "Climb_Reverse"=FALSE, "Low_Rocket"=FALSE, "Mid_Rocket"=FALSE, "High_Rocket"=FALSE, "Cargo_Ship"=FALSE, "Hatch_Floor"=FALSE, "Cargo_Floor"=FALSE, "HP_Hatch"=FALSE, "HP_Cargo"=FALSE, "Depot_Cargo"=FALSE, "Stow"=FALSE, "Set_Position"=enum."High_Rocket_Hatch_Panel", "Intake_Mode"=FALSE, "Climb_Distance"=0.0, "Level_Two"=FALSE, "Parameter_One"=0.0, "Parameter_Two"=0.0, "Parameter_Three"=0.0, "Step"=0, "Elevator_Notifier"=refnum, "Brake_State"=FALSE, "Shift_State"=FALSE}, "Climb_Notifier"={"Climb_Control_Type"=enum."No_Op", "Brake"=FALSE, "Manual_Climb_Up"=FALSE, "Manual_Drive_Forward"=FALSE, "Manual_Drive_Backward"=FALSE, "Manual_Climb_Down"=FALSE, "Climb_Advance"=FALSE, "Climb_Reverse"=FALSE, "Parameter_One"=0.0, "Parameter_Two"=0.0, "Parameter_Three"=0.0, "Step"=0, "Climb_Notifier"=refnum, "Climb_Distance"=0.0, "Level_Two"=FALSE, "Brake_State"=FALSE, "Toggle_Servo"=FALSE}, "Intake_Ball_Notifier"={"Intake_Ball_Control_Type"=enum."No_Op", "Manual_In"=FALSE, "Manual_Out"=FALSE, "Ball_In"=FALSE, "Ball_Out"=FALSE, "Parameter_One"=0.0, "Parameter_Two"=0.0, "Parameter_Three"=0.0, "Step"=0, "Ball_Notifier"=refnum}, "Intake_Disc_Notifier"={"Intake_Disc_Control_Type"=enum."No_Op", "Manual_Disc_Toggle"=FALSE, "Disc_Toggle"=FALSE, "Disc_Toggle_State"=FALSE, "Manual_Press_Toggle"=FALSE, "Disc_Press_State"=FALSE, "Press_Toggle"=FALSE, "Press_Pnuematic"=enum."Forward", "Disc_Pnuematic"=enum."Forward", "Disc_Notifier"=refnum, "Step"=0}, "Intake_Joint_Notifier"={"Intake_Joint_Control_Type"=enum."No_Op", "Manual_Joint_Up"=FALSE, "Manual_Joint_Down"=FALSE, "Low_Rocket"=FALSE, "Mid_Rocket"=FALSE, "High_Rocket"=FALSE, "Cargo_Ship"=FALSE, "Hatch_Floor"=FALSE, "Cargo_Floor"=FALSE, "HP_Hatch"=FALSE, "HP_Cargo"=FALSE, "Depot_Cargo"=FALSE, "Stow"=FALSE, "Intake_Mode"=FALSE, "Set Position"=enum."High_Rocket_Hatch_Panel", "Parameter_One"=0.0, "Parameter_Two"=0.0, "Parameter_Three"=0.0, "Step"=0, "Joint_Notifier"=refnum}} ("Robot Subsytems")) -> ()  [unwired: 1 out]
          n60 = in-place-cluster #6("Intake_Joint_Notifier"=w137) -> (w119:T10)
        }
        n61 = Enqueue Element(queue=w122, element=w119) -> (queue out=w118:refnum<queue>)  [unwired: 2 in, 2 out]
      }
      frame "Intake_Ball" {
        n62 = Number To Decimal String(number=w166) -> (decimal integer string=w169:string)  [unwired: 1 in]
        n63 = Concatenate Strings(w154, w169) -> (w168:string)
        n64 = Index Array(array=w167) -> (element #1=w146:string, element #2=w164:string, element #3=w144:string)  [unwired: 3 in]
        n65 = Scan From String(input string=w147, default 1="Intake_Ball_Control_Type") -> (output 1=w165:T2)  [unwired: 3 in, 3 out]
        n66 = Scan From String(input string=w164) -> (output 1=w163:dbl)  [unwired: 4 in, 3 out]
        n67 = Obtain Notifier(name (unnamed)=w168, notification data type=TRUE ("create if not found? (T)"), create if not found? (T)=TRUE) -> (notifier out=w153:refnum<notifier>)  [unwired: 1 in, 2 out]
        n68 = Scan From String(input string=w144, default 1=FALSE) -> (output 1=w151:bool)  [unwired: 3 in, 3 out]
        n69 = Scan From String(input string=w146) -> (output 1=w145:dbl)  [unwired: 4 in, 3 out]
        n70 = in-place {
          in-place-border: w153 -> [w176]
          in-place-border: w166 -> [w177]
          in-place-border: w165 -> [w175]
          in-place-border: w163 -> [w173]
          in-place-border: w145 -> [w174]
          n71 = in-place-cluster #7(T14 {"Intake_Ball_Control_Type"=enum."No_Op", "Manual_In"=FALSE, "Manual_Out"=FALSE, "Ball_In"=FALSE, "Ball_Out"=FALSE, "Parameter_One"=0.0, "Parameter_Two"=0.0, "Parameter_Three"=0.0, "Step"=0, "Ball_Notifier"=refnum} ("Intake_Ball_Notifier")) -> ()  [unwired: 5 out]
          n72 = in-place-cluster #7("Intake_Ball_Control_Type"=w175, "Parameter_One"=w174, "Parameter_Two"=w173, "Ball_Notifier"=w176, "Step"=w177) -> (w160:T14)
        }
        n73 = Bundle By Name(cluster=T9 {"Operation Notifier"=refnum, "Subsystem"="", "Concurrent"=FALSE} ("Queue Key Data"), "Operation Notifier"=w153, "Subsystem"=w154, "Concurrent"=w151) -> (w156:T9)
        n74 = Enqueue Element(queue=w157, element=w156) -> (queue out=w150:refnum<queue>)  [unwired: 2 in, 2 out]
        n75 = in-place {
          in-place-border: w160 -> [w172]
          n76 = in-place-cluster #8(T10 {"Drive Notifier"={"Drive Control List"=enum."No_Op", "Front/Back"=0.0, "Left/Right"=0.0, "Turn"=0.0, "Test_Joy_Y"=0.0, "Test_Joy_X"=0.0, "Set Wheel Encoder Positions"=FALSE, "Robotcentric"=FALSE, "Reset Gyro"=FALSE, "Rotate Front Right"=FALSE, "Rotate Front Left"=FALSE, "Rotate Back Right"=FALSE, "Rotate Back Left"=FALSE, "Write_Encoder_Positions"=FALSE, "Climb_Advance"=FALSE, "Parameter_One"=0.0, "Parameter_Two"=0.0, "Parameter_Three"=0.0, "Parameter_Four"=0.0, "Drive_Notifier"=refnum, "Step"=0, "Climb_Reverse"=FALSE, "Auto_Target"=FALSE}, "Elevator_Notifier"={"Elevator_Control_Type"=enum."No_Op", "Shift"=FALSE, "Brake"=FALSE, "Manual_Lift_Up"=FALSE, "Manual_Lift_Down"=FALSE, "Climb_Advance"=FALSE, "Climb_Reverse"=FALSE, "Low_Rocket"=FALSE, "Mid_Rocket"=FALSE, "High_Rocket"=FALSE, "Cargo_Ship"=FALSE, "Hatch_Floor"=FALSE, "Cargo_Floor"=FALSE, "HP_Hatch"=FALSE, "HP_Cargo"=FALSE, "Depot_Cargo"=FALSE, "Stow"=FALSE, "Set_Position"=enum."High_Rocket_Hatch_Panel", "Intake_Mode"=FALSE, "Climb_Distance"=0.0, "Level_Two"=FALSE, "Parameter_One"=0.0, "Parameter_Two"=0.0, "Parameter_Three"=0.0, "Step"=0, "Elevator_Notifier"=refnum, "Brake_State"=FALSE, "Shift_State"=FALSE}, "Climb_Notifier"={"Climb_Control_Type"=enum."No_Op", "Brake"=FALSE, "Manual_Climb_Up"=FALSE, "Manual_Drive_Forward"=FALSE, "Manual_Drive_Backward"=FALSE, "Manual_Climb_Down"=FALSE, "Climb_Advance"=FALSE, "Climb_Reverse"=FALSE, "Parameter_One"=0.0, "Parameter_Two"=0.0, "Parameter_Three"=0.0, "Step"=0, "Climb_Notifier"=refnum, "Climb_Distance"=0.0, "Level_Two"=FALSE, "Brake_State"=FALSE, "Toggle_Servo"=FALSE}, "Intake_Ball_Notifier"={"Intake_Ball_Control_Type"=enum."No_Op", "Manual_In"=FALSE, "Manual_Out"=FALSE, "Ball_In"=FALSE, "Ball_Out"=FALSE, "Parameter_One"=0.0, "Parameter_Two"=0.0, "Parameter_Three"=0.0, "Step"=0, "Ball_Notifier"=refnum}, "Intake_Disc_Notifier"={"Intake_Disc_Control_Type"=enum."No_Op", "Manual_Disc_Toggle"=FALSE, "Disc_Toggle"=FALSE, "Disc_Toggle_State"=FALSE, "Manual_Press_Toggle"=FALSE, "Disc_Press_State"=FALSE, "Press_Toggle"=FALSE, "Press_Pnuematic"=enum."Forward", "Disc_Pnuematic"=enum."Forward", "Disc_Notifier"=refnum, "Step"=0}, "Intake_Joint_Notifier"={"Intake_Joint_Control_Type"=enum."No_Op", "Manual_Joint_Up"=FALSE, "Manual_Joint_Down"=FALSE, "Low_Rocket"=FALSE, "Mid_Rocket"=FALSE, "High_Rocket"=FALSE, "Cargo_Ship"=FALSE, "Hatch_Floor"=FALSE, "Cargo_Floor"=FALSE, "HP_Hatch"=FALSE, "HP_Cargo"=FALSE, "Depot_Cargo"=FALSE, "Stow"=FALSE, "Intake_Mode"=FALSE, "Set Position"=enum."High_Rocket_Hatch_Panel", "Parameter_One"=0.0, "Parameter_Two"=0.0, "Parameter_Three"=0.0, "Step"=0, "Joint_Notifier"=refnum}} ("Robot Subsytems")) -> ()  [unwired: 1 out]
          n77 = in-place-cluster #8("Intake_Ball_Notifier"=w172) -> (w159:T10)
        }
        n78 = Enqueue Element(queue=w162, element=w159) -> (queue out=w158:refnum<queue>)  [unwired: 2 in, 2 out]
      }
      frame "Intake_Disc" {
        n79 = Number To Decimal String(number=w200) -> (decimal integer string=w202:string)  [unwired: 1 in]
        n80 = Concatenate Strings(w190, w202) -> (w201:string)
        n81 = Sort 1D Array(array=w180) -> (sorted array=w179:string[])
        n82 = Reverse 1D Array(array=w179) -> (reversed array=w178:string[])
        n83 = Index Array(array=w178, index=0) -> (element=w182:string)
        n84 = Scan From String(input string=w185, default 1="Intake_Disc_Control_Type") -> (output 1=w199:T1)  [unwired: 3 in, 3 out]
        n85 = Obtain Notifier(name (unnamed)=w201, notification data type=TRUE ("create if not found? (T)"), create if not found? (T)=TRUE) -> (notifier out=w189:refnum<notifier>)  [unwired: 1 in, 2 out]
        n86 = Scan From String(input string=w182, default 1=FALSE) -> (output 1=w187:bool)  [unwired: 3 in, 3 out]
        n87 = in-place {
          in-place-border: w189 -> [w207]
          in-place-border: w200 -> [w208]
          in-place-border: w199 -> [w206]
          n88 = in-place-cluster #9(T15 {"Intake_Disc_Control_Type"=enum."No_Op", "Manual_Disc_Toggle"=FALSE, "Disc_Toggle"=FALSE, "Disc_Toggle_State"=FALSE, "Manual_Press_Toggle"=FALSE, "Disc_Press_State"=FALSE, "Press_Toggle"=FALSE, "Press_Pnuematic"=enum."Forward", "Disc_Pnuematic"=enum."Forward", "Disc_Notifier"=refnum, "Step"=0} ("Intake_Disc_Notifier")) -> ()  [unwired: 3 out]
          n89 = in-place-cluster #9("Intake_Disc_Control_Type"=w206, "Disc_Notifier"=w207, "Step"=w208) -> (w196:T15)
        }
        n90 = Bundle By Name(cluster=T9 {"Operation Notifier"=refnum, "Subsystem"="", "Concurrent"=FALSE} ("Queue Key Data"), "Operation Notifier"=w189, "Subsystem"=w190, "Concurrent"=w187) -> (w192:T9)
        n91 = Enqueue Element(queue=w193, element=w192) -> (queue out=w186:refnum<queue>)  [unwired: 2 in, 2 out]
        n92 = in-place {
          in-place-border: w196 -> [w205]
          n93 = in-place-cluster #10(T10 {"Drive Notifier"={"Drive Control List"=enum."No_Op", "Front/Back"=0.0, "Left/Right"=0.0, "Turn"=0.0, "Test_Joy_Y"=0.0, "Test_Joy_X"=0.0, "Set Wheel Encoder Positions"=FALSE, "Robotcentric"=FALSE, "Reset Gyro"=FALSE, "Rotate Front Right"=FALSE, "Rotate Front Left"=FALSE, "Rotate Back Right"=FALSE, "Rotate Back Left"=FALSE, "Write_Encoder_Positions"=FALSE, "Climb_Advance"=FALSE, "Parameter_One"=0.0, "Parameter_Two"=0.0, "Parameter_Three"=0.0, "Parameter_Four"=0.0, "Drive_Notifier"=refnum, "Step"=0, "Climb_Reverse"=FALSE, "Auto_Target"=FALSE}, "Elevator_Notifier"={"Elevator_Control_Type"=enum."No_Op", "Shift"=FALSE, "Brake"=FALSE, "Manual_Lift_Up"=FALSE, "Manual_Lift_Down"=FALSE, "Climb_Advance"=FALSE, "Climb_Reverse"=FALSE, "Low_Rocket"=FALSE, "Mid_Rocket"=FALSE, "High_Rocket"=FALSE, "Cargo_Ship"=FALSE, "Hatch_Floor"=FALSE, "Cargo_Floor"=FALSE, "HP_Hatch"=FALSE, "HP_Cargo"=FALSE, "Depot_Cargo"=FALSE, "Stow"=FALSE, "Set_Position"=enum."High_Rocket_Hatch_Panel", "Intake_Mode"=FALSE, "Climb_Distance"=0.0, "Level_Two"=FALSE, "Parameter_One"=0.0, "Parameter_Two"=0.0, "Parameter_Three"=0.0, "Step"=0, "Elevator_Notifier"=refnum, "Brake_State"=FALSE, "Shift_State"=FALSE}, "Climb_Notifier"={"Climb_Control_Type"=enum."No_Op", "Brake"=FALSE, "Manual_Climb_Up"=FALSE, "Manual_Drive_Forward"=FALSE, "Manual_Drive_Backward"=FALSE, "Manual_Climb_Down"=FALSE, "Climb_Advance"=FALSE, "Climb_Reverse"=FALSE, "Parameter_One"=0.0, "Parameter_Two"=0.0, "Parameter_Three"=0.0, "Step"=0, "Climb_Notifier"=refnum, "Climb_Distance"=0.0, "Level_Two"=FALSE, "Brake_State"=FALSE, "Toggle_Servo"=FALSE}, "Intake_Ball_Notifier"={"Intake_Ball_Control_Type"=enum."No_Op", "Manual_In"=FALSE, "Manual_Out"=FALSE, "Ball_In"=FALSE, "Ball_Out"=FALSE, "Parameter_One"=0.0, "Parameter_Two"=0.0, "Parameter_Three"=0.0, "Step"=0, "Ball_Notifier"=refnum}, "Intake_Disc_Notifier"={"Intake_Disc_Control_Type"=enum."No_Op", "Manual_Disc_Toggle"=FALSE, "Disc_Toggle"=FALSE, "Disc_Toggle_State"=FALSE, "Manual_Press_Toggle"=FALSE, "Disc_Press_State"=FALSE, "Press_Toggle"=FALSE, "Press_Pnuematic"=enum."Forward", "Disc_Pnuematic"=enum."Forward", "Disc_Notifier"=refnum, "Step"=0}, "Intake_Joint_Notifier"={"Intake_Joint_Control_Type"=enum."No_Op", "Manual_Joint_Up"=FALSE, "Manual_Joint_Down"=FALSE, "Low_Rocket"=FALSE, "Mid_Rocket"=FALSE, "High_Rocket"=FALSE, "Cargo_Ship"=FALSE, "Hatch_Floor"=FALSE, "Cargo_Floor"=FALSE, "HP_Hatch"=FALSE, "HP_Cargo"=FALSE, "Depot_Cargo"=FALSE, "Stow"=FALSE, "Intake_Mode"=FALSE, "Set Position"=enum."High_Rocket_Hatch_Panel", "Parameter_One"=0.0, "Parameter_Two"=0.0, "Parameter_Three"=0.0, "Step"=0, "Joint_Notifier"=refnum}} ("Robot Subsytems")) -> ()  [unwired: 1 out]
          n94 = in-place-cluster #10("Intake_Disc_Notifier"=w205) -> (w195:T10)
        }
        n95 = Enqueue Element(queue=w198, element=w195) -> (queue out=w194:refnum<queue>)  [unwired: 2 in, 2 out]
      }
      frame "Climb" {
        n96 = Number To Decimal String(number=w232) -> (decimal integer string=w236:string)  [unwired: 1 in]
        n97 = Concatenate Strings(w217, w236) -> (w235:string)
        n98 = Index Array(array=w209) -> (element #1=w231:string, element #2=w229:string, element #3=w226:string, element #4=w214:string)  [unwired: 4 in]
        n99 = Scan From String(input string=w234, default 1="Climb_Control_Type") -> (output 1=w233:T7)  [unwired: 3 in, 3 out]
        n100 = Scan From String(input string=w231) -> (output 1=w230:dbl)  [unwired: 4 in, 3 out]
        n101 = Scan From String(input string=w229) -> (output 1=w228:dbl)  [unwired: 4 in, 3 out]
        n102 = Scan From String(input string=w226) -> (output 1=w227:dbl)  [unwired: 4 in, 3 out]
        n103 = Scan From String(input string=w214, default 1=FALSE) -> (output 1=w213:bool)  [unwired: 3 in, 3 out]
        n104 = Obtain Notifier(name (unnamed)=w235, notification data type=TRUE ("create if not found? (T)"), create if not found? (T)=TRUE) -> (notifier out=w216:refnum<notifier>)  [unwired: 1 in, 2 out]
        n105 = in-place {
          in-place-border: w233 -> [w245]
          in-place-border: w216 -> [w244]
          in-place-border: w232 -> [w243]
          in-place-border: w230 -> [w242]
          in-place-border: w228 -> [w241]
          in-place-border: w227 -> [w240]
          n106 = in-place-cluster #11(T13 {"Climb_Control_Type"=enum."No_Op", "Brake"=FALSE, "Manual_Climb_Up"=FALSE, "Manual_Drive_Forward"=FALSE, "Manual_Drive_Backward"=FALSE, "Manual_Climb_Down"=FALSE, "Climb_Advance"=FALSE, "Climb_Reverse"=FALSE, "Parameter_One"=0.0, "Parameter_Two"=0.0, "Parameter_Three"=0.0, "Step"=0, "Climb_Notifier"=refnum, "Climb_Distance"=0.0, "Level_Two"=FALSE, "Brake_State"=FALSE, "Toggle_Servo"=FALSE} ("Climb_Notifier")) -> ()  [unwired: 6 out]
          n107 = in-place-cluster #11("Climb_Control_Type"=w245, "Parameter_One"=w242, "Parameter_Two"=w241, "Parameter_Three"=w240, "Climb_Notifier"=w244, "Step"=w243) -> (w223:T13)
        }
        n108 = Bundle By Name(cluster=T9 {"Operation Notifier"=refnum, "Subsystem"="", "Concurrent"=FALSE} ("Queue Key Data"), "Operation Notifier"=w216, "Subsystem"=w217, "Concurrent"=w213) -> (w219:T9)
        n109 = Enqueue Element(queue=w220, element=w219) -> (queue out=w212:refnum<queue>)  [unwired: 2 in, 2 out]
        n110 = in-place {
          in-place-border: w223 -> [w239]
          n111 = in-place-cluster #12(T10 {"Drive Notifier"={"Drive Control List"=enum."No_Op", "Front/Back"=0.0, "Left/Right"=0.0, "Turn"=0.0, "Test_Joy_Y"=0.0, "Test_Joy_X"=0.0, "Set Wheel Encoder Positions"=FALSE, "Robotcentric"=FALSE, "Reset Gyro"=FALSE, "Rotate Front Right"=FALSE, "Rotate Front Left"=FALSE, "Rotate Back Right"=FALSE, "Rotate Back Left"=FALSE, "Write_Encoder_Positions"=FALSE, "Climb_Advance"=FALSE, "Parameter_One"=0.0, "Parameter_Two"=0.0, "Parameter_Three"=0.0, "Parameter_Four"=0.0, "Drive_Notifier"=refnum, "Step"=0, "Climb_Reverse"=FALSE, "Auto_Target"=FALSE}, "Elevator_Notifier"={"Elevator_Control_Type"=enum."No_Op", "Shift"=FALSE, "Brake"=FALSE, "Manual_Lift_Up"=FALSE, "Manual_Lift_Down"=FALSE, "Climb_Advance"=FALSE, "Climb_Reverse"=FALSE, "Low_Rocket"=FALSE, "Mid_Rocket"=FALSE, "High_Rocket"=FALSE, "Cargo_Ship"=FALSE, "Hatch_Floor"=FALSE, "Cargo_Floor"=FALSE, "HP_Hatch"=FALSE, "HP_Cargo"=FALSE, "Depot_Cargo"=FALSE, "Stow"=FALSE, "Set_Position"=enum."High_Rocket_Hatch_Panel", "Intake_Mode"=FALSE, "Climb_Distance"=0.0, "Level_Two"=FALSE, "Parameter_One"=0.0, "Parameter_Two"=0.0, "Parameter_Three"=0.0, "Step"=0, "Elevator_Notifier"=refnum, "Brake_State"=FALSE, "Shift_State"=FALSE}, "Climb_Notifier"={"Climb_Control_Type"=enum."No_Op", "Brake"=FALSE, "Manual_Climb_Up"=FALSE, "Manual_Drive_Forward"=FALSE, "Manual_Drive_Backward"=FALSE, "Manual_Climb_Down"=FALSE, "Climb_Advance"=FALSE, "Climb_Reverse"=FALSE, "Parameter_One"=0.0, "Parameter_Two"=0.0, "Parameter_Three"=0.0, "Step"=0, "Climb_Notifier"=refnum, "Climb_Distance"=0.0, "Level_Two"=FALSE, "Brake_State"=FALSE, "Toggle_Servo"=FALSE}, "Intake_Ball_Notifier"={"Intake_Ball_Control_Type"=enum."No_Op", "Manual_In"=FALSE, "Manual_Out"=FALSE, "Ball_In"=FALSE, "Ball_Out"=FALSE, "Parameter_One"=0.0, "Parameter_Two"=0.0, "Parameter_Three"=0.0, "Step"=0, "Ball_Notifier"=refnum}, "Intake_Disc_Notifier"={"Intake_Disc_Control_Type"=enum."No_Op", "Manual_Disc_Toggle"=FALSE, "Disc_Toggle"=FALSE, "Disc_Toggle_State"=FALSE, "Manual_Press_Toggle"=FALSE, "Disc_Press_State"=FALSE, "Press_Toggle"=FALSE, "Press_Pnuematic"=enum."Forward", "Disc_Pnuematic"=enum."Forward", "Disc_Notifier"=refnum, "Step"=0}, "Intake_Joint_Notifier"={"Intake_Joint_Control_Type"=enum."No_Op", "Manual_Joint_Up"=FALSE, "Manual_Joint_Down"=FALSE, "Low_Rocket"=FALSE, "Mid_Rocket"=FALSE, "High_Rocket"=FALSE, "Cargo_Ship"=FALSE, "Hatch_Floor"=FALSE, "Cargo_Floor"=FALSE, "HP_Hatch"=FALSE, "HP_Cargo"=FALSE, "Depot_Cargo"=FALSE, "Stow"=FALSE, "Intake_Mode"=FALSE, "Set Position"=enum."High_Rocket_Hatch_Panel", "Parameter_One"=0.0, "Parameter_Two"=0.0, "Parameter_Three"=0.0, "Step"=0, "Joint_Notifier"=refnum}} ("Robot Subsytems")) -> ()  [unwired: 1 out]
          n112 = in-place-cluster #12("Climb_Notifier"=w239) -> (w222:T10)
        }
        n113 = Enqueue Element(queue=w225, element=w222) -> (queue out=w221:refnum<queue>)  [unwired: 2 in, 2 out]
      }
    }
  }
  "Queue_Key" <- w3
  "Autonomous_Queue" <- w2
  "errror out" <- "error in"
